vi "Parse Session (Rx-UDP).vi"(8 "error in":errorcluster, 11 "node in":refnum<k20>) -> (0 "error out":errorcluster, 3 "tx udp session out":T1={"VerificationMode"=0, "Bag"=0, "Jitter"=1, "MaxFrameLength"=0, "MaxSkew"=1, "VLBufSize"=1, "FilterMode"=1, "FilterPosition"=1, "Padding"=0, "FilterMask"=0, "FilterData"=0, "MinFrameLength"=0, "VlId"=0, "VLRange"=0} {"FilterMode" items=["FDX_TX_FRAME_DLY_A"=0, "FDX_TX_FRAME_DLY_B"=1, "FDX_TX_FRAME_BOTH "=3, "FDX_TX_FRAME_ONLY_A"=4, "FDX_TX_FRAME_ONLY_B "=5]; "MaxSkew" format="%.0b"; "VerificationMode" items=["FDX_RX_VL_CHECK_ENA_DEFAULT"=65535, "FDX_RX_VL_CHECK_REDMAM"=16, "DX_RX_VL_CHECK_TRAFIC"=8, "FDX_RX_VL_CHECK_FRAMESIZE"=4, "FDX_RX_VL_CHECK_SNINTEG"=2, "FDX_RX_VL_CHECK_INVPAC"=1, "FDX_RX_VL_CHECK_DISA"=0]})   [LabVIEW 2020, in "AIM ARINC 664 Import.lvlib"]
uses:
  AIM ARINC 664 Import.lvlib
  _typedefs/rx_udp_setup.ctl
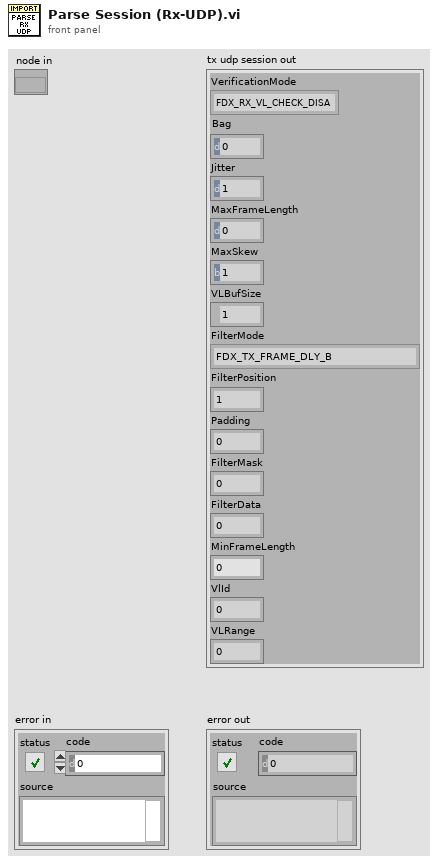
[diagram p1: front panel]
types:
  T1 = typedef "AIM ARINC 664 Import.lvlib/rx_udp_setup.ctl" = cluster{"VerificationMode":u32, "Bag":u32, "Jitter":u32, "MaxFrameLength":u32, "MaxSkew":u32, "VLBufSize":u32, "FilterMode":u32, "FilterPosition":u32, "Padding":u32, "FilterMask":u32, "FilterData":u32, "MinFrameLength":u32, "VlId":u16, "VLRange":u32}
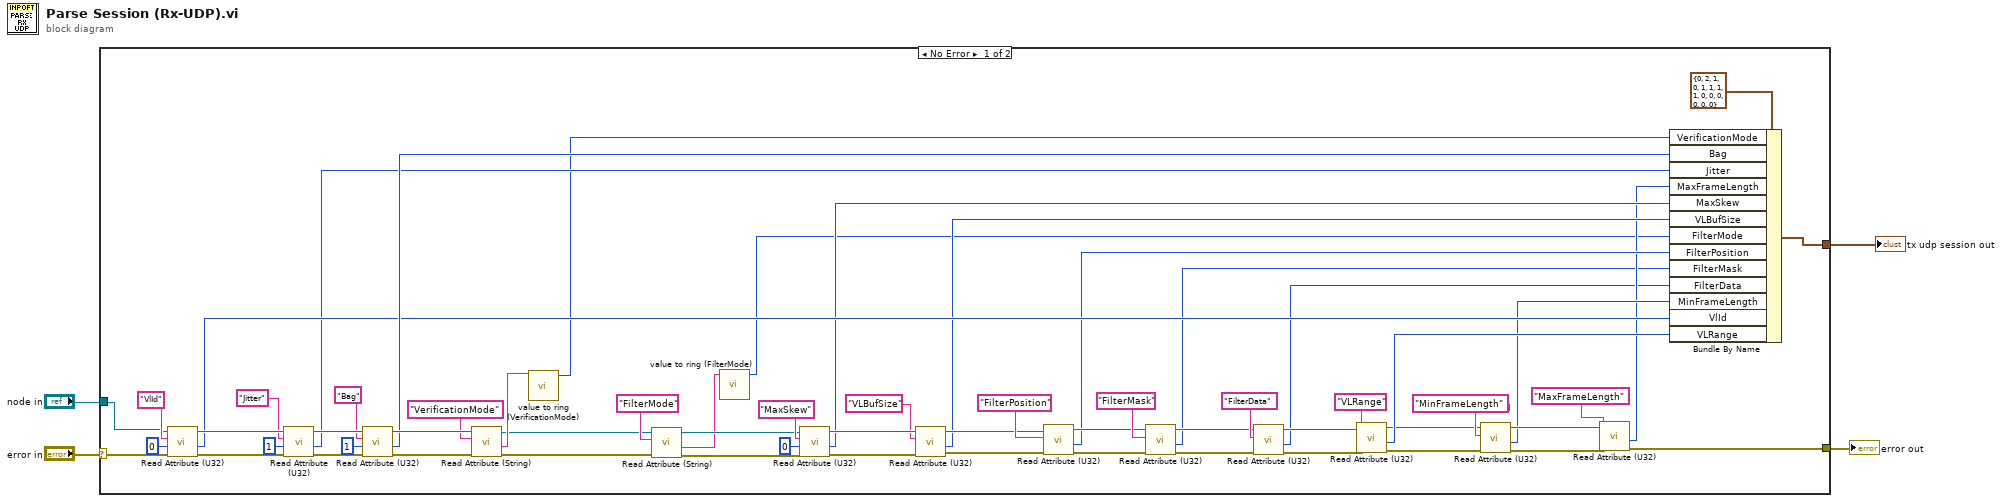
[diagram p0: block diagram]
diagram:
  n1 = case shown="No Error" "error in" {
    selector: "error in" -> [w53 w66]
    tunnel: "node in" -> [w52 _]
    tunnel: [w16 w66] -> w3
    tunnel: [w54 _] -> w1
    frame No Error {
      n2 = call "Read Attribute (U32).vi"("error in"=w53, "default"=u32 0, "Attribute Name"="VlId" ("Tag Name"), "node in"=w52) -> ("error out"=w61:errorcluster, "value"=w34:u32, "node out"=w60:refnum<k20>)  [unwired: 5 in]
      n3 = call "Read Attribute (U32).vi"("error in"=w61, "default"=u32 1, "Attribute Name"="Jitter" ("Tag Name"), "node in"=w60) -> ("error out"=w63:errorcluster, "value"=w33:u32, "node out"=w62:refnum<k20>)  [unwired: 5 in]
      n4 = call "Read Attribute (U32).vi"("error in"=w63, "default"=u32 1, "Attribute Name"="Bag" ("Tag Name"), "node in"=w62) -> ("error out"=w65:errorcluster, "value"=w35:u32, "node out"=w64:refnum<k20>)  [unwired: 5 in]
      n5 = call "Read Attribute (String).vi"("error in"=w65, "Attribute Name"="VerificationMode" ("Tag Name"), "node in"=w64) -> ("error out"=w14:errorcluster, "value"=w32:string, "node out"=w13:refnum<k20>)  [unwired: 6 in]
      n6 = call "value to ring (VerificationMode).vi"("value"=w32) -> ("VerificationMode"=w31:u32)  [unwired: 10 in]
      n7 = call "Read Attribute (String).vi"("error in"=w14, "Attribute Name"="FilterMode" ("Tag Name"), "node in"=w13) -> ("error out"=w12:errorcluster, "value"=w10:string, "node out"=w11:refnum<k20>)  [unwired: 6 in]
      n8 = call "value to ring (FilterMode).vi"("value"=w10) -> ("FilterMode"=w9:u32)  [unwired: 10 in]
      n9 = call "Read Attribute (U32).vi"("error in"=w12, "default"=u32 0, "Attribute Name"="MaxSkew" ("Tag Name"), "node in"=w11) -> ("error out"=w51:errorcluster, "value"=w30:u32, "node out"=w50:refnum<k20>)  [unwired: 5 in]
      n10 = call "Read Attribute (U32).vi"("error in"=w51, "Attribute Name"="VLBufSize" ("Tag Name"), "node in"=w50) -> ("error out"=w43:errorcluster, "value"=w29:u32, "node out"=w44:refnum<k20>)  [unwired: 6 in]
      n11 = call "Read Attribute (U32).vi"("error in"=w43, "Attribute Name"="FilterPosition" ("Tag Name"), "node in"=w44) -> ("error out"=w42:errorcluster, "value"=w28:u32, "node out"=w46:refnum<k20>)  [unwired: 6 in]
      n12 = call "Read Attribute (U32).vi"("error in"=w42, "Attribute Name"="FilterMask" ("Tag Name"), "node in"=w46) -> ("error out"=w36:errorcluster, "value"=w18:u32, "node out"=w37:refnum<k20>)  [unwired: 6 in]
      n13 = call "Read Attribute (U32).vi"("error in"=w36, "Attribute Name"="FilterData" ("Tag Name"), "node in"=w37) -> ("error out"=w38:errorcluster, "value"=w17:u32, "node out"=w39:refnum<k20>)  [unwired: 6 in]
      n14 = call "Read Attribute (U32).vi"("error in"=w38, "Attribute Name"="VLRange" ("Tag Name"), "node in"=w39) -> ("error out"=w23:errorcluster, "value"=w27:u32, "node out"=w21:refnum<k20>)  [unwired: 6 in]
      n15 = call "Read Attribute (U32).vi"("error in"=w23, "Attribute Name"="MinFrameLength" ("Tag Name"), "node in"=w21) -> ("error out"=w26:errorcluster, "value"=w20:u32, "node out"=w25:refnum<k20>)  [unwired: 6 in]
      n16 = call "Read Attribute (U32).vi"("error in"=w26, "Attribute Name"="MaxFrameLength" ("Tag Name"), "node in"=w25) -> ("error out"=w16:errorcluster, "value"=w19:u32)  [unwired: 6 in, 1 out]
      n17 = Bundle By Name(cluster=T1 {"VerificationMode"=0, "Bag"=2, "Jitter"=1, "MaxFrameLength"=0, "MaxSkew"=1, "VLBufSize"=1, "FilterMode"=1, "FilterPosition"=1, "Padding"=0, "FilterMask"=0, "FilterData"=0, "MinFrameLength"=0, "VlId"=0, "VLRange"=0} ("boardSetup"), "VerificationMode"=w31, "Bag"=w35, "Jitter"=w33, "MaxFrameLength"=w19, "MaxSkew"=w30, "VLBufSize"=w29, "FilterMode"=w9, "FilterPosition"=w28, "FilterMask"=w18, "FilterData"=w17, "MinFrameLength"=w20, "VlId"=w34, "VLRange"=w27) -> (w54:T1)
    }
    frame Error {
    }
  }
  "error out" <- w3
  "tx udp session out" <- w1
